vi "Verify Waveform And XY Plots.vi"(2 "[user-specified font]":T1={"Font Name:"="Current Font", "Size"=36, "Strikeout?"=FALSE, "Italic?"=FALSE, "Underline?"=FALSE, "Outline?"=TRUE, "Shadow?"=TRUE, "Bold?"=TRUE}, 3 "desired font(Application)":T2(ring), 4 "Text To Draw":string) -> (0 "xy plot Out":picture, 1 "waveform plot Out":picture)   [LabVIEW 2010]
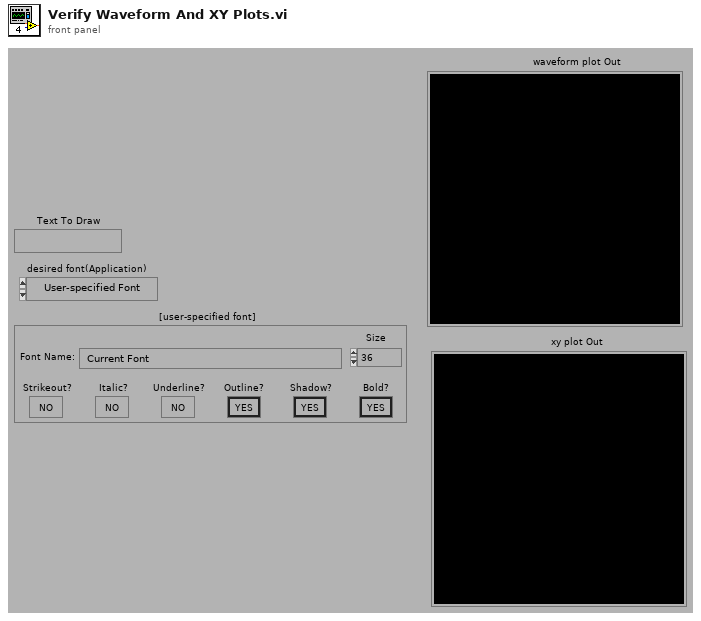
[diagram p1: front panel]
types:
  T1 = cluster{"Font Name:":string, "Size":i16, "Strikeout?":bool, "Italic?":bool, "Underline?":bool, "Outline?":bool, "Shadow?":bool, "Bold?":bool}
  T2 = enum16{"User-specified Font", "Application Font", "System Font", "Dialog Font"}
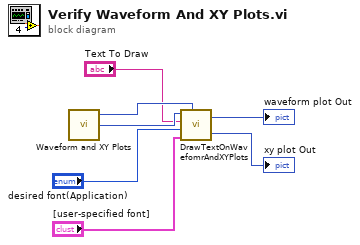
[diagram p0: block diagram]
diagram:
  n1 = call "Waveform and XY Plots.vi"() -> ("xy plot"=w7:picture, "waveform plot"=w6:picture)  [unwired: 4 out]
  n2 = call "DrawTextOnWavefomrAndXYPlots.vi"("xy plot In"=w7, "Text To Draw"="Text To Draw", "desired font(Application)"="desired font(Application)", "[user-specified font]"="[user-specified font]", "waveform plot In"=w6) -> ("waveform plot Out"=→"waveform plot Out":picture, "xy plot Out"=→"xy plot Out":picture)
